vi "WriteMoxa12.vi"(0 "DATA ISMA 4":dbl, 1 "DATA ISMA 3":dbl, 2 "DATA ISMA 2":dbl, 3 "DATA ISMA 1":dbl, 4 "PORT ISMA 4":dbl, 5 "DATA LAUDA 2":dbl, 6 "PORT ISMA 3":dbl, 7 "DATA LAUDA 1":dbl, 8 "PORT ISMA 2":dbl, 9 "PORT ISMA 1":dbl, 10 "PORT LAUDA 2":dbl, 11 "PORT LAUDA 1":dbl) -> ()   [LabVIEW 2017]
uses:
  BERTTA.dll
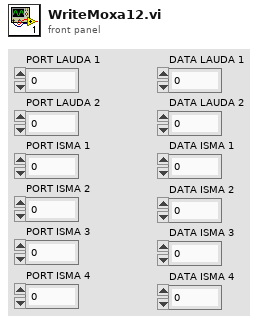
[diagram p1: front panel]
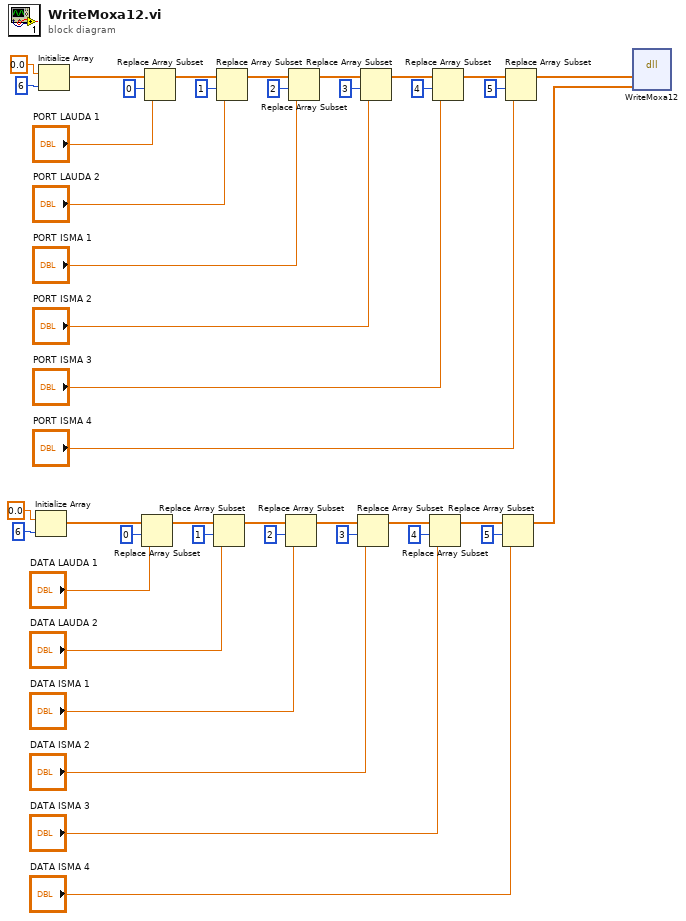
[diagram p0: block diagram]
diagram:
  n1 = Initialize Array(0.0 ("element"), 6 ("dimension size")) -> (w19:dbl[])
  n2 = Initialize Array(0.0 ("element"), 6 ("dimension size")) -> (w40:dbl[])
  n3 = Replace Array Subset(array=w19, new element="DATA LAUDA 1", index=0) -> (w18:dbl[])
  n4 = Replace Array Subset(array=w40, new element="PORT LAUDA 1", index=0) -> (w39:dbl[])
  n5 = Replace Array Subset(array=w18, new element="DATA LAUDA 2", index=1) -> (w17:dbl[])
  n6 = Replace Array Subset(array=w39, new element="PORT LAUDA 2", index=1) -> (w38:dbl[])
  n7 = Replace Array Subset(array=w17, new element="DATA ISMA 1", index=2) -> (w16:dbl[])
  n8 = Replace Array Subset(array=w38, new element="PORT ISMA 1", index=2) -> (w37:dbl[])
  n9 = Replace Array Subset(array=w16, new element="DATA ISMA 2", index=3) -> (w15:dbl[])
  n10 = Replace Array Subset(array=w37, new element="PORT ISMA 2", index=3) -> (w36:dbl[])
  n11 = Replace Array Subset(array=w15, new element="DATA ISMA 3", index=4) -> (w14:dbl[])
  n12 = Replace Array Subset(array=w36, new element="PORT ISMA 3", index=4) -> (w35:dbl[])
  n13 = Replace Array Subset(array=w14, new element="DATA ISMA 4", index=5) -> (w1:dbl[])
  n14 = Replace Array Subset(array=w35, new element="PORT ISMA 4", index=5) -> (w34:dbl[])
  n15 = dll-call lib="C:/Users/shresplab/OneDrive - Kemira Oyj/Documents/GitHub/Bertta/BERTTA/x64/Debug/BERTTA.dll" fn="WriteMoxa12"("ports"=w34, "params"=w1) -> ()  [unwired: 6 in, 2 out]
